vi "逐点滤波.vi"(1 "Forward Coefficients":dbl[](array[numeric]) caption="前向系数", 2 "输入x":dbl caption="原始信号x" format="%0.2f") -> (0 "Filtered x":dbl caption="滤波后的x" format="%0.2f")   [LabVIEW 2018]
uses:
  <vilib>/Analysis/3filter.llb/Filter Passband Type.ctl
  <vilib>/Utility/file.llb/Read Delimited Spreadsheet (DBL).vi
  <vilib>/ptbypt/NI_PtbyPt.lvlib
  <vilib>/Analysis/NI_AALBase.lvlib
panel:
  in  "file path (dialog if empty) 3":path caption="文件路径 （空时为对话框）"
  in  "file path (dialog if empty) 2":path caption="文件路径 （空时为对话框）"
  in  "file path (dialog if empty)":path caption="文件路径 （空时为对话框）"
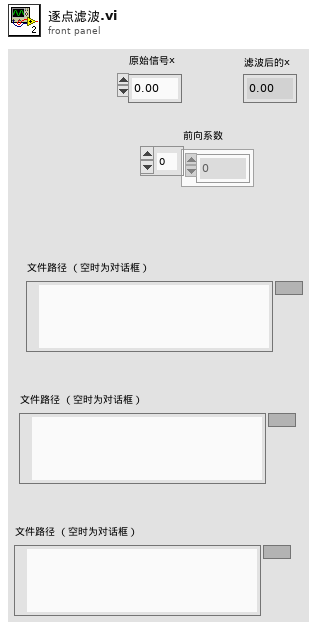
[diagram p1: front panel]
types:
  T1 = typedef "NI_AALBase.lvlib/Filter Passband Type.ctl" = enum32{"Lowpass", "Highpass", "Bandpass", "Bandstop"}
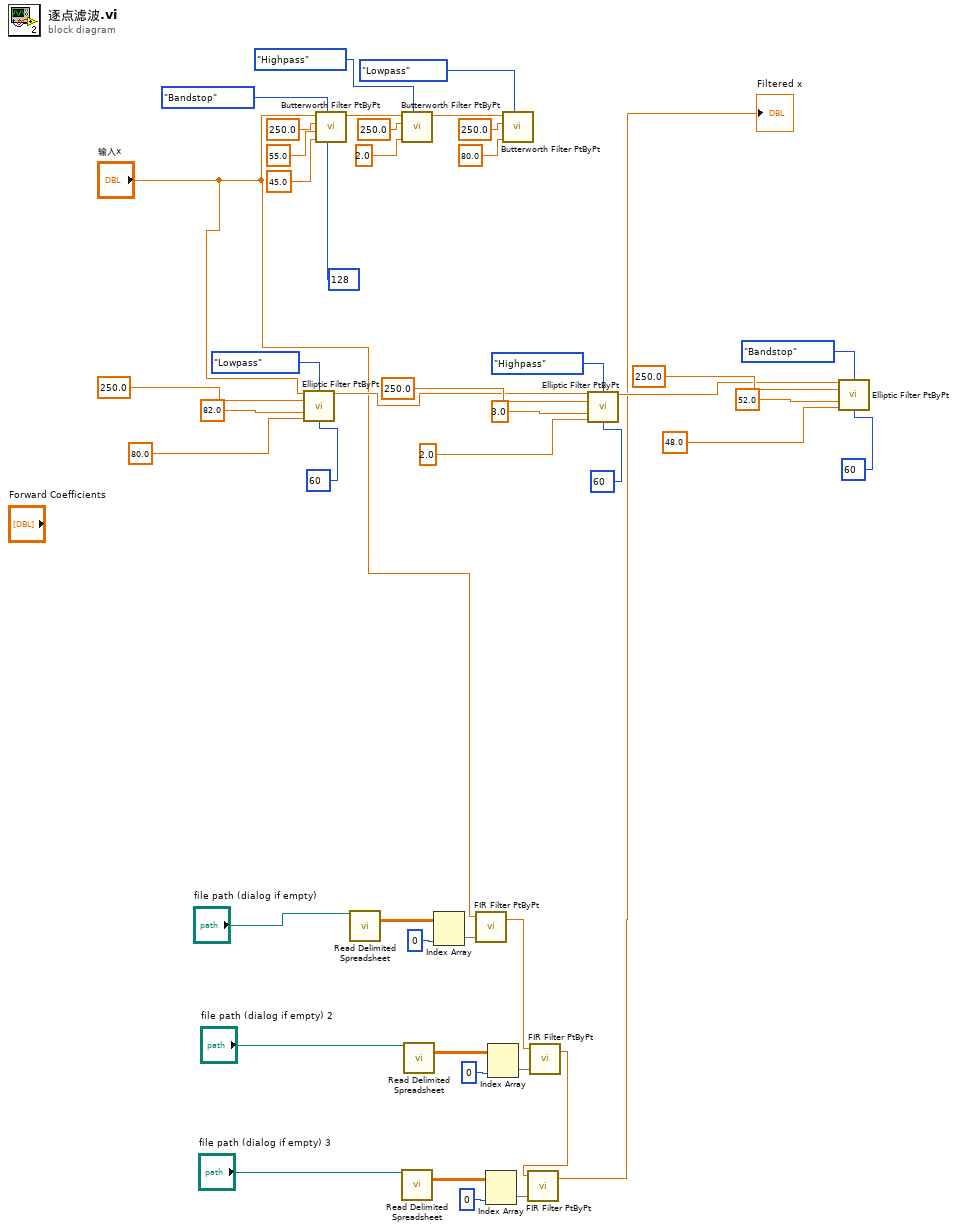
[diagram p0: block diagram]
diagram:
  n1 = call <vilib>:"Elliptic Filter PtByPt.vi"("x"="输入x", "filter type"=Filter_Passband_Type."Lowpass", "sampling freq: fs"=250.0, "high cutoff freq: fh"=82.0, "low cutoff freq: fl"=80.0, "order"=60) -> ("Filtered x"=w18:dbl)  [unwired: 8 in, 1 out]
  n2 = call <vilib>:"Butterworth Filter PtByPt.vi"("order"=128, "filter type"=Filter_Passband_Type."Bandstop", "low cutoff freq: fl"=45.0, "high cutoff freq: fh"=55.0, "sampling freq: fs"=250.0, "x"="输入x") -> ("Filtered x"=w36:dbl)  [unwired: 3 in, 1 out]
  n3 = call-poly <vilib>:"Read Delimited Spreadsheet.vi"("file path (dialog if empty)"="file path (dialog if empty)") -> ("all rows"=w14:dbl[][])  [unwired: 9 in, 5 out]
  n4 = call <vilib>:"Butterworth Filter PtByPt.vi"("filter type"=Filter_Passband_Type."Highpass", "low cutoff freq: fl"=2.0, "sampling freq: fs"=250.0, "x"=w36) -> ("Filtered x"=w35:dbl)  [unwired: 5 in, 1 out]
  n5 = call-poly <vilib>:"Read Delimited Spreadsheet.vi"("file path (dialog if empty)"="file path (dialog if empty) 3") -> ("all rows"=w6:dbl[][])  [unwired: 9 in, 5 out]
  n6 = call-poly <vilib>:"Read Delimited Spreadsheet.vi"("file path (dialog if empty)"="file path (dialog if empty) 2") -> ("all rows"=w10:dbl[][])  [unwired: 9 in, 5 out]
  n7 = Index Array(array=w14, index (col)=0 ("禁用的索引 (列)")) -> (element=w12:dbl[])  [unwired: 1 in]
  n8 = call <vilib>:"FIR Filter PtByPt.vi"("Forward Coefficients"=w12, "x"="输入x") -> ("Filtered x"=w2:dbl)  [unwired: 2 in, 1 out]
  n9 = Index Array(array=w6, index (col)=0 ("禁用的索引 (列)")) -> (element=w4:dbl[])  [unwired: 1 in]
  n10 = Index Array(array=w10, index (col)=0 ("禁用的索引 (列)")) -> (element=w8:dbl[])  [unwired: 1 in]
  n11 = call <vilib>:"Butterworth Filter PtByPt.vi"("filter type"=Filter_Passband_Type."Lowpass", "low cutoff freq: fl"=80.0, "sampling freq: fs"=250.0, "x"=w35) -> ()  [unwired: 5 in, 2 out]
  n12 = call <vilib>:"FIR Filter PtByPt.vi"("Forward Coefficients"=w8, "x"=w2) -> ("Filtered x"=w1:dbl)  [unwired: 2 in, 1 out]
  n13 = call <vilib>:"FIR Filter PtByPt.vi"("Forward Coefficients"=w4, "x"=w1) -> ("Filtered x"=→"Filtered x":dbl)  [unwired: 2 in, 1 out]
  n14 = call <vilib>:"Elliptic Filter PtByPt.vi"("x"=w18, "filter type"=Filter_Passband_Type."Highpass", "sampling freq: fs"=250.0, "high cutoff freq: fh"=3.0, "low cutoff freq: fl"=2.0, "order"=60) -> ("Filtered x"=w17:dbl)  [unwired: 8 in, 1 out]
  n15 = call <vilib>:"Elliptic Filter PtByPt.vi"("x"=w17, "filter type"=Filter_Passband_Type."Bandstop", "sampling freq: fs"=250.0, "high cutoff freq: fh"=52.0, "low cutoff freq: fl"=48.0, "order"=60) -> ()  [unwired: 8 in, 2 out]
